vi "VISA_Read_2CH.vi"() -> ()   [LabVIEW 2019]
uses:
  <vilib>/Instr/_visa.llb/VISA Configure Serial Port (Instr).vi
panel:
  out "Status Serial":errorcluster
  in  "Stop Read":bool
  in  "Start Read":bool
  in  "baud rate (9600)":u32=115200
  in  "data bits (8)":u8=8 min=5 max=8 step=1
  in  "VISA resource name":refnum<visa-resource-name>
  out "Buffer Array":dbl[][](array[numeric])
  out "Read Buffer":string
  out "Status Read":errorcluster
  out "Buffer Plot":dbl[][](graph)
  # "Conversão Para Inteiro"
  # "Controle da porta Serial USB"
  # "Controle da Leitura"
  # "Resultado da Leitura"
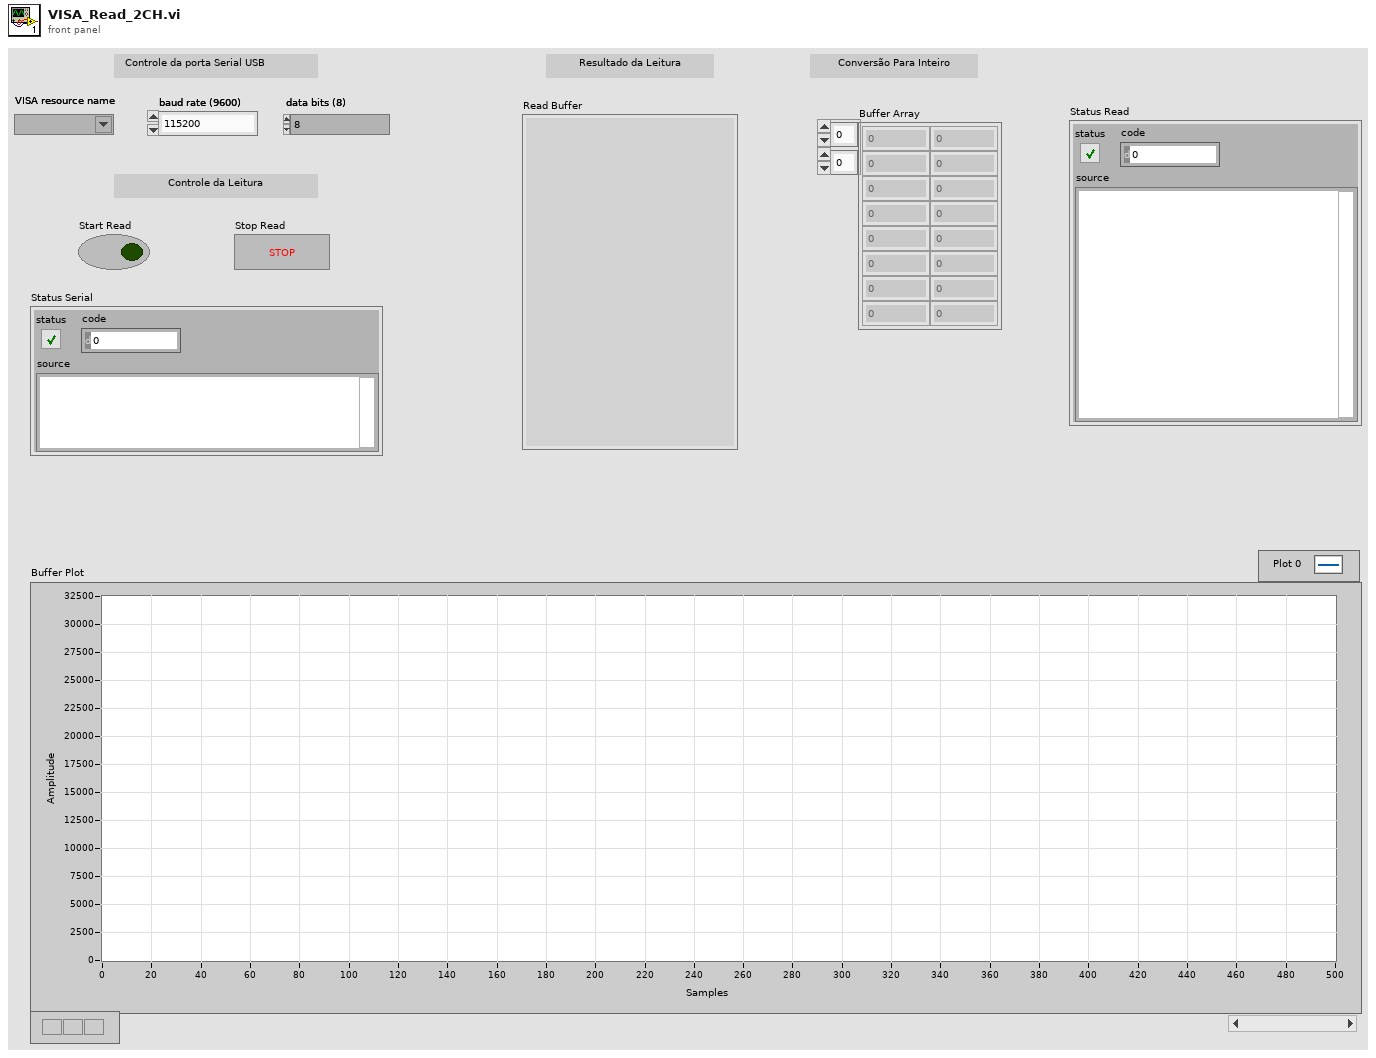
[diagram p1: front panel]
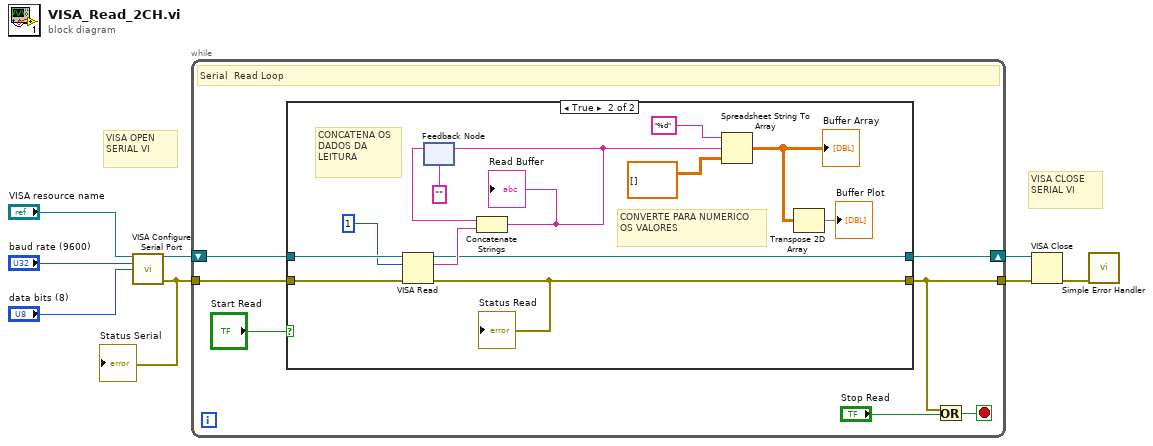
[diagram p0: block diagram]
diagram:
  # "VISA CLOSE SERIAL VI"
  # "VISA OPEN SERIAL VI"
  n1 = call-poly "VISA Configure Serial Port"("VISA resource name"="VISA resource name", "baud rate (9600)"="baud rate (9600)", "data bits (8)"="data bits (8)") -> ("VISA resource name out"=w7:refnum<visa-resource-name>, "error out"=w4:errorcluster)  [unwired: 11 in]
  "Status Serial" <- w4
  n2 = while {
    tunnel: w4 -> [w15]
    tunnel: [w13] -> w8
    shift-right: [w11] -> w6
    shift-left: w7 -> [w12]
    stop <- w14 stop-if-true
    # "Serial  Read Loop"
    n3 = case shown="True" "Start Read" {
      tunnel: w15 -> [w16 w30]
      tunnel: [w16 w29] -> w13
      tunnel: w12 -> [w17 w25]
      tunnel: [w17 w24] -> w11
      frame False {
      }
      frame True {
        # "CONVERTE PARA NUMERICO OS VALORES"
        # "CONCATENA OS DADOS DA LEITURA"
        n4 = VISA Read(VISA resource name=w25, byte count=u32 1, error in (no error)=w30) -> (VISA resource name out=w24:refnum<visa-resource-name>, read buffer=w28:string, error out=w29:errorcluster)  [unwired: 1 out]
        "Status Read" <- w29
        n5 = feedback #1("") -> (w27:string)
        n6 = Concatenate Strings(w27, w28) -> (w23:string)
        "Read Buffer" <- w23
        n7 = feedback-in #1(w23) -> ()
        n8 = Spreadsheet String To Array(format string="%d", spreadsheet string=w23, array type (2D Dbl)=dbl[][] []) -> (array=w19:dbl[][])  [unwired: 1 in]
        "Buffer Array" <- w19
        n9 = Transpose 2D Array(2D array=w19) -> (transposed array=→"Buffer Plot":dbl[][])
      }
    }
    n10 = Or(x=w13, y="Stop Read") -> (x .or. y?=w14:bool)
  }
  n11 = VISA Close(VISA resource name=w6, error in (no error)=w8) -> (error out=w5:errorcluster)
  n12 = call <vilib>:"Simple Error Handler.vi"("error in (no error)"=w5) -> ()  [unwired: 4 in, 5 out]
